vi "Destroy.vi"(8 "Error In":errorcluster, 11 "Display In":refnum<class "Neopixel - Host.lvclass">) -> (0 "Error Out":errorcluster)   [LabVIEW 2021, in "Neopixel - Host.lvclass"]
uses:
  Neopixel - Host.lvclass
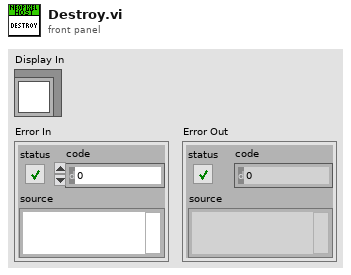
[diagram p1: front panel]
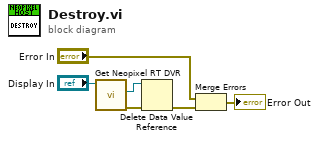
[diagram p0: block diagram]
diagram:
  n1 = call "Get Neopixel RT DVR.vi"("Display In"="Display In") -> ("Error Out"=w5:errorcluster, "DVR"=w4:refnum<data-value>)  [unwired: 8 in, 1 out]
  n2 = Delete Data Value Reference(data value reference=w4, error in=w5) -> (error out=w1:errorcluster)  [unwired: 1 out]
  n3 = Merge Errors("Error In", w1) -> (→"Error Out":errorcluster)
